vi "Test Parse lvproj with Class with Virtual Folder.vi"(11 "Test Case In":refnum<class "Parsing XML.lvclass">) -> (0 "error out":errorcluster, 3 "Test Case Out":refnum<class "Parsing XML.lvclass">)   [LabVIEW 2020, in "Parsing XML.lvclass"]
uses:
  Parsing XML.lvclass
  Parsing XML.lvclass/Parsing XML.ctl
  4993e8ee-a06a-463a-9684-69129f64d5ce.vi
  source/VI Properties Editor.lvlib
  source/Classes/Item/Item.lvclass
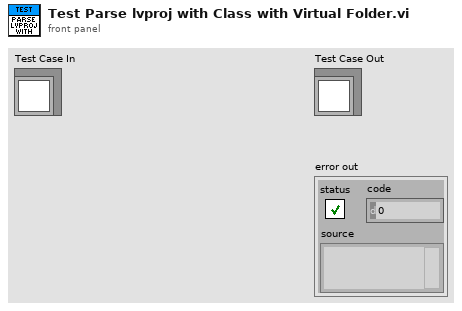
[diagram p1: front panel]
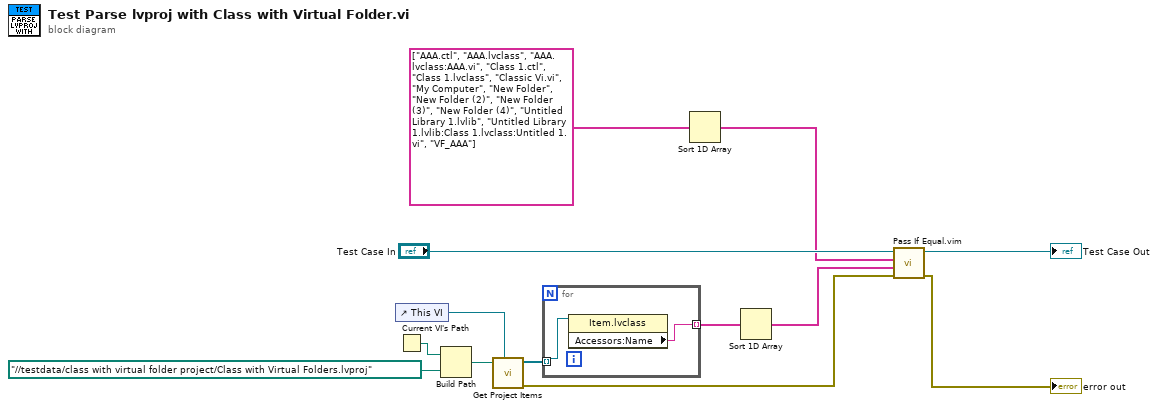
[diagram p0: block diagram]
diagram:
  n1 = control-ref of="This VI"() -> (w1:refnum<vi>)
  n2 = Current VI's Path() -> (path=w10:path)
  n3 = Build Path(base path=w10, name or relative path=path "../../testdata/class with virtual folder project/Class with Virtual Folders.lvproj") -> (appended path=w7:path)
  n4 = call "Get Project Items.vi"("Calling VI Ref"=w1, "Path"=w7) -> ("error out"=w9:errorcluster, "Items Data"=w8:refnum<class "Item.lvclass">[])  [unwired: 7 in, 1 out]
  n5 = for {
    tunnel: w8 -> [w15] mode=indexing
    tunnel: [w14] -> w3 mode=indexing
    n6 = property class="Item.lvclass"(reference=w15) -> ("Accessors:Name"=w14:string)  [unwired: 1 in, 2 out]
  }
  n7 = Sort 1D Array(array=string[] ["AAA.ctl", "AAA.lvclass", "AAA.lvclass:AAA.vi", "Class 1.ctl", "Class 1.lvclass", "Classic Vi.vi", "My Computer", "New Folder", "New Folder (2)", "New Folder (3)", "New Folder (4)", "Untitled Library 1.lvlib", "Untitled Library 1.lvlib:Class 1.lvclass:Untitled 1.vi", "VF_AAA"] ("sorted array")) -> (sorted array=w6:string[])
  n8 = Sort 1D Array(array=w3) -> (sorted array=w5:string[])
  n9 = call "Pass If Equal.vim"("error in (no error)"=w9, "Actual"=w5, "Expected"=w6, "LUnit Test Case In"="Test Case In") -> ("error out"=→"error out":errorcluster, "LUnit Test Case Out"=→"Test Case Out":refnum<class "Parsing XML.lvclass">)  [unwired: 6 in]
